vi "反控参数变更.vi"(11 "设置参数":T1(ring)=enum."CODMn") -> ()   [LabVIEW 2022 SP3, in "斯坦道通用流路CODmn.lvlib"]
panel:
  in  "错误输入（无错误）":errorcluster
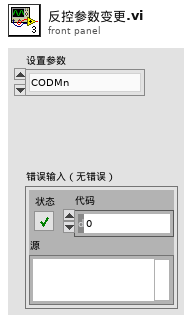
[diagram p1: front panel]
types:
  T1 = enum16{"", "CODMn", "PH", "氨氮", "总氮", "总磷", "CODCr", "电导率", "水温", "溶解氧", "浊度", "叶绿素", "藻密度", "ORP"}
  T2 = typedef "斯坦道通用流路CODmn.lvlib/量程模式.ctl" = enum32{"H", "L", "AUTO"}
  T3 = typedef "操作日志字段定义.ctl" = cluster{"时间":timestamp, "参数":string, "日志信息":string, "流程参数":string}
  T4 = cluster{"水样测试量程模式":enum16{"H", "L", "AUTO"}, "空白核查量程模式":enum16{"H", "L", "AUTO"}, "跨度核查量程模式":enum16{"H", "L", "AUTO"}, "加标回收量程模式":enum16{"H", "L", "AUTO"}, "标样核查量程模式":enum16{"H", "L", "AUTO"}}
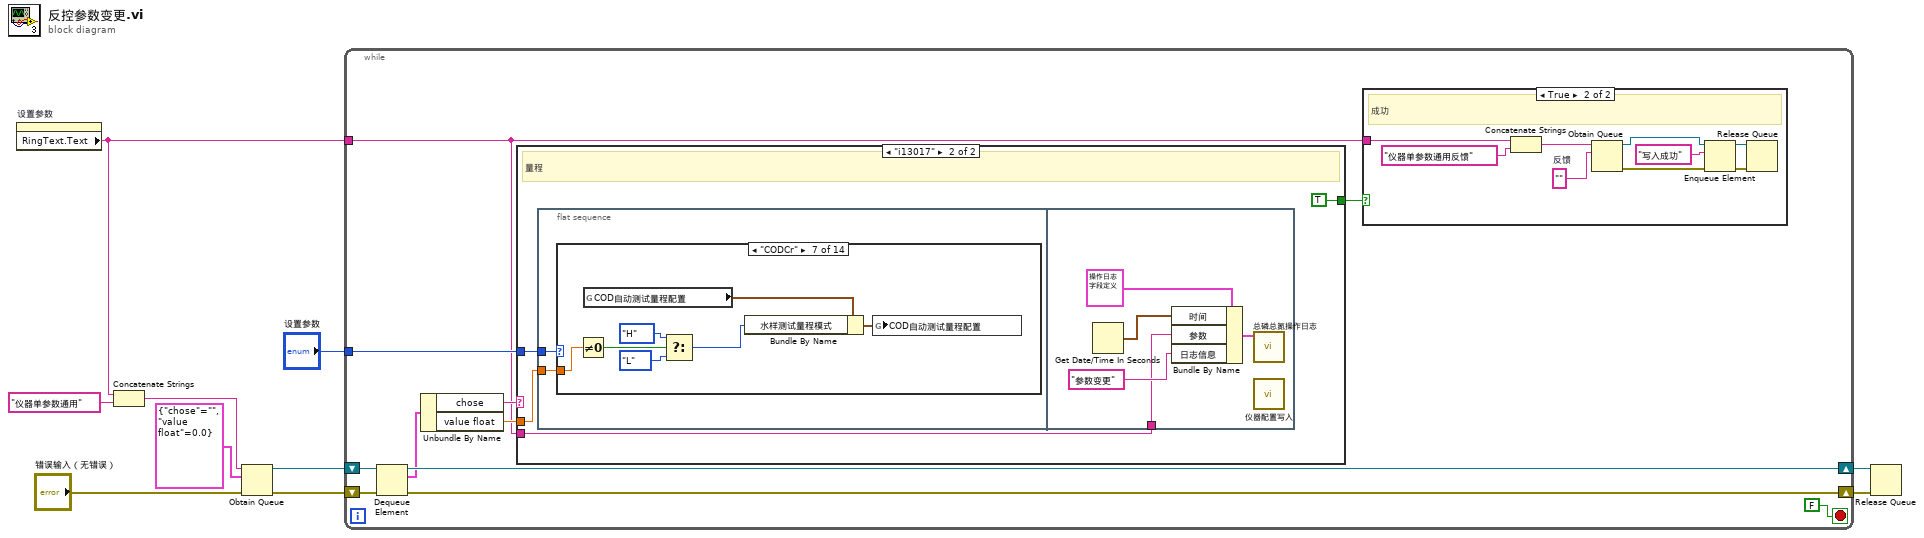
[diagram p0: block diagram]
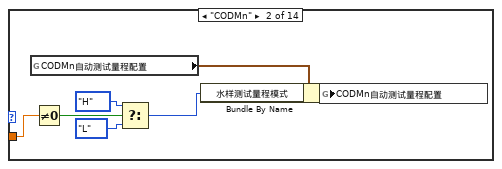
[diagram p5: hidden frame]
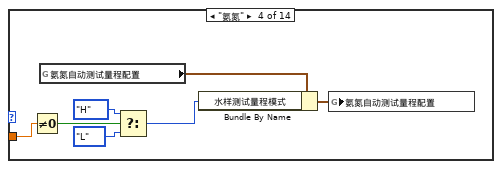
[diagram p7: hidden frame]
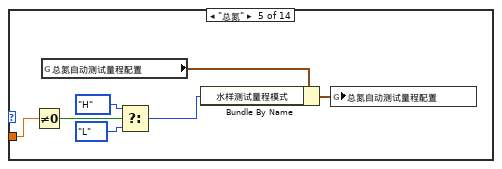
[diagram p8: hidden frame]
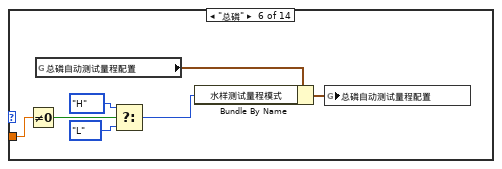
[diagram p9: hidden frame]
diagram:
  n1 = property on="设置参数" class="Enum (strict)"() -> ("RingText.Text"=w2:string)  [unwired: 2 in, 2 out]
  n2 = Concatenate Strings(w2, "仪器单参数通用" ("名称（未命名）")) -> (w7:string)
  n3 = Obtain Queue(name (unnamed)=w7, element data type=cluster{"chose":string, "value float":dbl} {"chose"="", "value float"=0.0}, error in (no error)="错误输入（无错误）") -> (queue out=w6:refnum<queue>, error out=w5:errorcluster)  [unwired: 2 in, 1 out]
  n4 = while {
    shift-right: [w19] -> w4
    shift-left: w6 -> [w21]
    shift-right: [w18] -> w3
    shift-left: w5 -> [w20]
    tunnel: w2 -> [w11]
    tunnel: "设置参数" -> [w12]
    stop <- FALSE stop-if-true
    n5 = Dequeue Element(queue=w21, error in (no error)=w20) -> (queue out=w19:refnum<queue>, element=w16:cluster{"chose":string, "value float":dbl}, error out=w18:errorcluster)  [unwired: 1 in, 1 out]
    n6 = Unbundle By Name(w16) -> ("chose"=w15:string, "value float"=w13:dbl)
    n7 = case shown="\"i13017\"" w15 {
      tunnel: w13 -> [_ w32]
      tunnel: [_ TRUE] -> w14
      tunnel: w12 -> [_ w33]
      tunnel: w11 -> [_ w31]
      frame "假", Default {
      }
      frame "i13017" {
        # "量程"
        n8 = flat-sequence {
          tunnel: w33 -> [w36]
          tunnel: w32 -> [w35]
          tunnel: w31 -> [w72]
          frame #0 {
            n9 = case shown="\"CODCr\"" w36 {
              tunnel: w35 -> [_ w37 _ w44 w51 w58 w65 _ _ _ _ _ _ _]
              frame "", Default {
              }
              frame "CODMn" {
                n10 = global read "总磷总氮断电保存全局变量.vi" "CODMn自动测试量程配置"() -> (w43:T4)
                n11 = Not Equal To 0?(x=w37) -> (x != 0?=w41:bool)
                n12 = Select(t=量程模式."H" ("水样测试量程模式"), s=w41, f=量程模式."L" ("水样测试量程模式")) -> (s? t:f=w38:T2)
                n13 = Bundle By Name(cluster=w43, "水样测试量程模式"=w38) -> (w42:T4)
                n14 = global write "总磷总氮断电保存全局变量.vi" "CODMn自动测试量程配置"(w42) -> ()
              }
              frame "PH" {
              }
              frame "氨氮" {
                n15 = Not Equal To 0?(x=w44) -> (x != 0?=w48:bool)
                n16 = global read "总磷总氮断电保存全局变量.vi" "氨氮自动测试量程配置"() -> (w50:T4)
                n17 = Select(t=量程模式."H" ("水样测试量程模式"), s=w48, f=量程模式."L" ("水样测试量程模式")) -> (s? t:f=w45:T2)
                n18 = Bundle By Name(cluster=w50, "水样测试量程模式"=w45) -> (w49:T4)
                n19 = global write "总磷总氮断电保存全局变量.vi" "氨氮自动测试量程配置"(w49) -> ()
              }
              frame "总氮" {
                n20 = Not Equal To 0?(x=w51) -> (x != 0?=w55:bool)
                n21 = global read "总磷总氮断电保存全局变量.vi" "总氮自动测试量程配置"() -> (w57:T4)
                n22 = Select(t=量程模式."H" ("水样测试量程模式"), s=w55, f=量程模式."L" ("水样测试量程模式")) -> (s? t:f=w52:T2)
                n23 = Bundle By Name(cluster=w57, "水样测试量程模式"=w52) -> (w56:T4)
                n24 = global write "总磷总氮断电保存全局变量.vi" "总氮自动测试量程配置"(w56) -> ()
              }
              frame "总磷" {
                n25 = Not Equal To 0?(x=w58) -> (x != 0?=w62:bool)
                n26 = global read "总磷总氮断电保存全局变量.vi" "总磷自动测试量程配置"() -> (w64:T4)
                n27 = Select(t=量程模式."H" ("水样测试量程模式"), s=w62, f=量程模式."L" ("水样测试量程模式")) -> (s? t:f=w59:T2)
                n28 = Bundle By Name(cluster=w64, "水样测试量程模式"=w59) -> (w63:T4)
                n29 = global write "总磷总氮断电保存全局变量.vi" "总磷自动测试量程配置"(w63) -> ()
              }
              frame "CODCr" {
                n30 = Not Equal To 0?(x=w65) -> (x != 0?=w69:bool)
                n31 = global read "总磷总氮断电保存全局变量.vi" "COD自动测试量程配置"() -> (w71:T4)
                n32 = Select(t=量程模式."H" ("水样测试量程模式"), s=w69, f=量程模式."L" ("水样测试量程模式")) -> (s? t:f=w66:T2)
                n33 = Bundle By Name(cluster=w71, "水样测试量程模式"=w66) -> (w70:T4)
                n34 = global write "总磷总氮断电保存全局变量.vi" "COD自动测试量程配置"(w70) -> ()
              }
              frame "电导率" {
              }
              frame "水温" {
              }
              frame "溶解氧" {
              }
              frame "浊度" {
              }
              frame "叶绿素" {
              }
              frame "藻密度" {
              }
              frame "ORP" {
              }
            }
          }
          frame #1 {
            n35 = Get Date/Time In Seconds() -> (seconds since 1Jan1904=w75:timestamp)
            n36 = Bundle By Name(cluster=T3 {"时间"=timestamp(0 s since 1904-01-01), "参数"="", "日志信息"="", "流程参数"=""} ("data in"), "时间"=w75, "参数"=w72, "日志信息"="参数变更") -> (w74:T3)
            n37 = call "总磷总氮操作日志.vi"("data in"=w74) -> ()  [unwired: 10 in, 1 out]
            n38 = call "仪器配置写入.vi"() -> ()  [unwired: 11 in, 1 out]
          }
        }
      }
    }
    n39 = case shown="True" w14 {
      tunnel: w11 -> [_ w29]
      frame False {
      }
      frame True {
        w24 = ""  # 反馈
        # "成功"
        n40 = Concatenate Strings(w29, "仪器单参数通用反馈" ("名称（未命名）")) -> (w23:string)
        n41 = Obtain Queue(name (unnamed)=w23, element data type=w24) -> (queue out=w25:refnum<queue>, error out=w26:errorcluster)  [unwired: 3 in, 1 out]
        n42 = Enqueue Element(queue=w25, element="写入成功" ("元素"), error in (no error)=w26) -> (queue out=w28:refnum<queue>, error out=w27:errorcluster)  [unwired: 1 in, 1 out]
        n43 = Release Queue(queue=w28, error in (no error)=w27) -> ()  [unwired: 1 in, 3 out]
      }
    }
  }
  n44 = Release Queue(queue=w4, error in (no error)=w3) -> ()  [unwired: 1 in, 3 out]
